vi "Find Ballard ARINC-429 Custom Devices.vi"(8 "error in":errorcluster, 11 "target":refnum<k24>) -> (0 "error out":errorcluster, 3 "Ballard ARINC-429 custom devices":u64[](array[numeric]))   [LabVIEW 2020, in "Communication Bus Template Scripting.lvlib"]
uses:
  Communication Bus Template Scripting.lvlib
  NationalInstruments.VeriStand.SystemDefinitionAPI
  Constants.vi
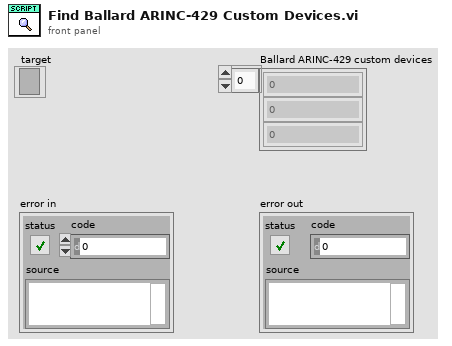
[diagram p1: front panel]
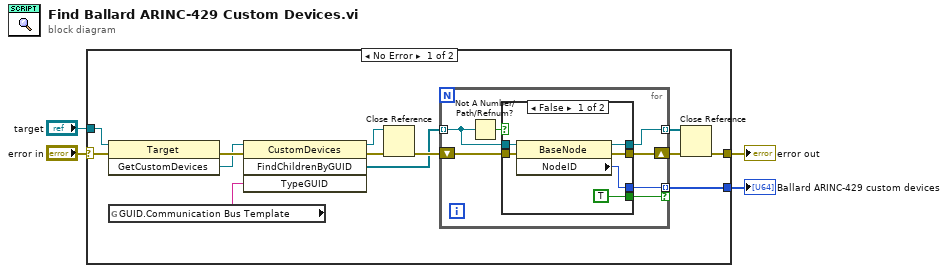
[diagram p0: block diagram]
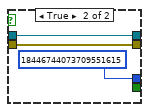
[diagram p2: hidden frame]
diagram:
  n1 = case shown="No Error" "error in" {
    selector: "error in" -> [w6 w34]
    tunnel: "target" -> [w10 _]
    tunnel: [w7 _] -> w3
    tunnel: [w5 w34] -> w1
    frame No Error {
      n2 = invoke class="Target" method="GetCustomDevices"(reference=w10, error in=w6) -> (error out=w17:errorcluster, "GetCustomDevices"=w16:refnum<k24>)  [unwired: 1 in, 1 out]
      n3 = global read "Constants.vi" "GUID.Communication Bus Template"() -> (w9:string)
      n4 = invoke class="CustomDevices" method="FindChildrenByGUID"(reference=w16, error in=w17, "TypeGUID"=w9) -> (reference out=w15:refnum<k24>, error out=w14:errorcluster, "FindChildrenByGUID"=w8:refnum<k24>[])  [unwired: 1 in, 1 out]
      n5 = Close Reference(reference=w15, error in (no error)=w14) -> (error out=w13:errorcluster)
      n6 = for {
        shift-right: [w22] -> w11
        shift-left: w13 -> [w24]
        tunnel: w8 -> [w21] mode=indexing
        tunnel: [w23] -> w12 mode=indexing
        tunnel: [w19] -> w7 mode=indexing if=w18
        n7 = Not A Number/Path/Refnum?(number/path/refnum=w21) -> (NaN/Path/Refnum?=w20:bool)
        n8 = case shown="False" w20 {
          tunnel: [w26 w33] -> w22
          tunnel: w24 -> [w28 w33]
          tunnel: w21 -> [w30 w32]
          tunnel: [w29 u64 18446744073709551615 ("NodeID")] -> w19
          tunnel: [w27 w32] -> w23
          tunnel: [TRUE _] -> w18
          frame False {
            n9 = property class="BaseNode"(reference=w30, error in=w28) -> (reference out=w27:refnum<k24>, error out=w26:errorcluster, "NodeID"=w29:u64)
          }
          frame True {
          }
        }
      }
      n10 = Close Reference(reference=w12, error in (no error)=w11) -> (error out=w5:errorcluster)
    }
    frame Error {
    }
  }
  "Ballard ARINC-429 custom devices" <- w3
  "error out" <- w1
